vi "InitDone.vi"(8 "error in (no error)":errorcluster, 10 "Variant":variant, 11 "TranslationStageUI.lvclass":refnum<class "TranslationStageUI.lvclass">) -> (0 "error out":errorcluster, 3 "TranslationStageUI.lvclass":refnum<class "TranslationStageUI.lvclass">)   [LabVIEW 2023, in "TranslationStageUI.lvclass"]
uses:
  TranslationStageUI.lvclass
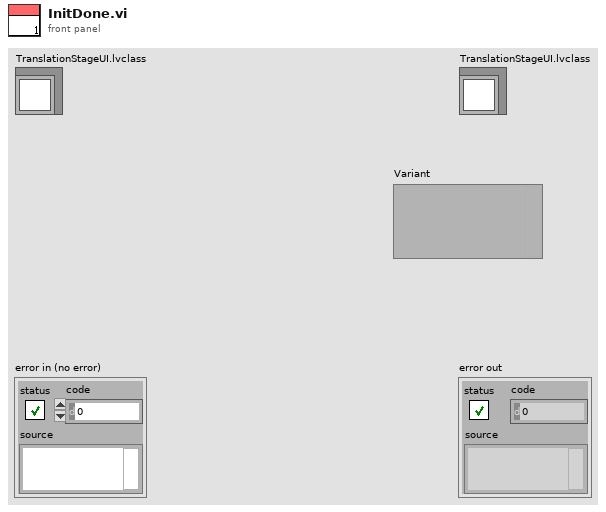
[diagram p1: front panel]
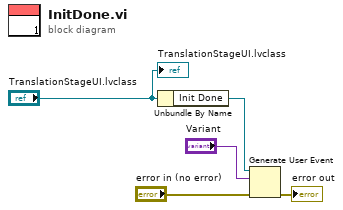
[diagram p0: block diagram]
diagram:
  n1 = Unbundle By Name("TranslationStageUI.lvclass") -> ("Init Done"=w3:refnum<user-event>)
  n2 = Generate User Event(user event=w3, event data cluster="Variant", error in="error in (no error)") -> (error out=→"error out":errorcluster)  [unwired: 1 in, 1 out]
  "TranslationStageUI.lvclass" <- "TranslationStageUI.lvclass"
